vi "Core Handle Error.vi"(8 "error in (no error)":errorcluster, 11 "CIFTemplateNode in":refnum<class "CIFCorePlugin.lvclass">) -> (0 "error out":errorcluster, 3 "CIFTemplateNode out":refnum<class "CIFCorePlugin.lvclass">)   [LabVIEW 2021, in "CIFCorePlugin.lvclass"]
uses:
  CIFCorePlugin.lvclass
  CIFCorePlugin.lvclass/CIFCorePlugin.ctl
  Typedef/Energized States.ctl
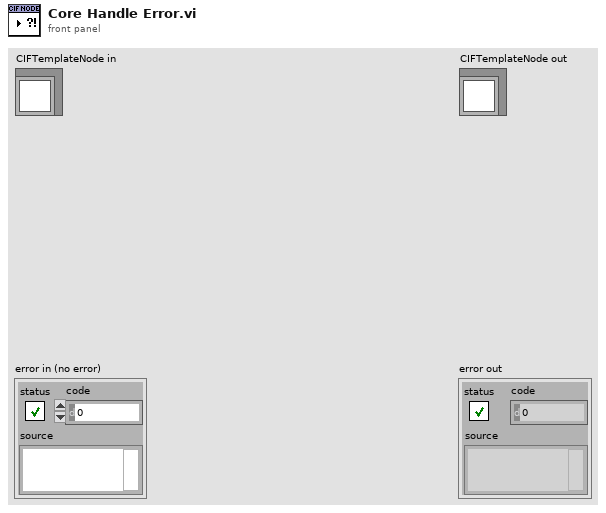
[diagram p1: front panel]
types:
  T1 = typedef "CIFCorePlugin.lvclass/Energized States.ctl" = enum16{"Listen", "Prepare", "Execute", "Housekeep", "Cleanup", "Destroy"}
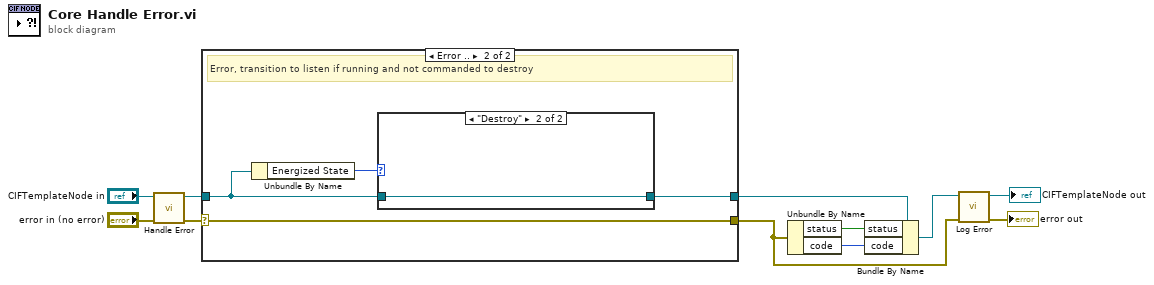
[diagram p0: block diagram]
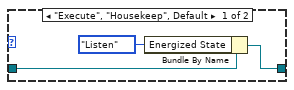
[diagram p3: hidden frame]
diagram:
  n1 = call-dynamic "Handle Error.vi"("error in (no error)"="error in (no error)", "CIFTemplateNode in"="CIFTemplateNode in") -> ("error out"=w8:errorcluster, "CIFTemplateNode out"=w10:refnum<class "CIFCorePlugin.lvclass">)  [unwired: 8 in]
  n2 = case shown="Error .." w8 {
    selector: w8 -> [w12 w14]
    tunnel: [w13 w16] -> w7
    tunnel: w10 -> [w13 w15]
    tunnel: [w12 w14] -> w3
    frame No Error {
      # "Warning, Only log."
    }
    frame Error {
      # "Error, transition to listen if running and not commanded to destroy"
      n3 = Unbundle By Name(w15) -> ("Energized State"=w17:T1)
      n4 = case shown="\"Destroy\"" w17 {
        tunnel: [w19 w21] -> w16
        tunnel: w15 -> [w20 w21]
        frame "Execute", "Housekeep", Default {
          n5 = Bundle By Name(cluster=w20, "Energized State"=Energized_States."Listen") -> (w19:refnum<class "CIFCorePlugin.lvclass">)
        }
        frame "Destroy" {
        }
      }
    }
  }
  n6 = Unbundle By Name(w3) -> ("status"=w6:bool, "code"=w5:i32)
  n7 = Bundle By Name(cluster=w7, "status"=w6, "code"=w5) -> (w4:refnum<class "CIFCorePlugin.lvclass">)
  n8 = call "Log Error.vi"("error in (no error)"=w3, "CIFCorePlugin in"=w4) -> ("error out"=→"error out":errorcluster, "CIFCorePlugin out"=→"CIFTemplateNode out":refnum<class "CIFCorePlugin.lvclass">)  [unwired: 8 in]
